vi "Initialize.vi"(8 "error in":errorcluster, 11 "cPAS Subject in":refnum<class "cPAS Subject.lvclass">) -> (0 "error out":errorcluster, 2 "DVR":refnum<data-value>, 3 "cPAS Subject out":refnum<class "cPAS Subject.lvclass">)   [LabVIEW 2015, in "cPAS Subject.lvclass"]
uses:
  cPAS Subject.lvclass
  Reusable/Data/Data.lvclass
  Data/cPAS Data.lvclass
  Reusable/Observer/Data Subject.lvclass/Data Subject.ctl
  Reusable/Observer/Data Subject.lvclass
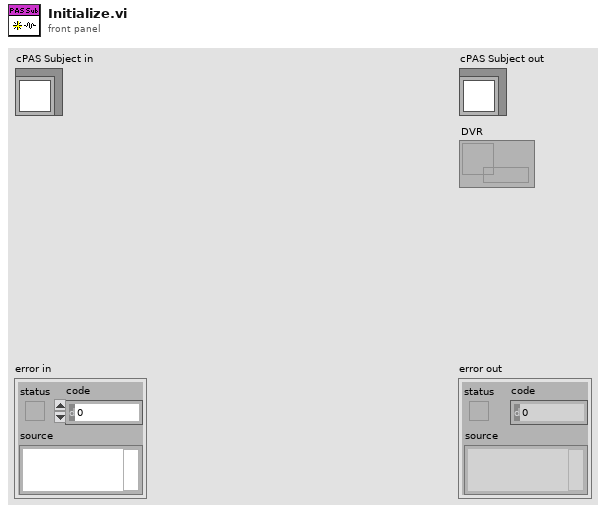
[diagram p1: front panel]
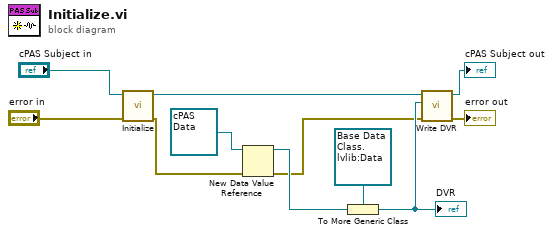
[diagram p0: block diagram]
diagram:
  n1 = call-parent "Initialize.vi"("error in"="error in", "Data Subject in"="cPAS Subject in") -> ("error out"=w8:errorcluster, "Data Subject out"=w7:refnum<class "cPAS Subject.lvclass">)  [unwired: 7 in, 1 out]
  n2 = New Data Value Reference(data value=refnum<class "cPAS Data.lvclass"> refnum ("cPAS Data"), error in=w8) -> (data value reference=w5:refnum<data-value>, error out=w1:errorcluster)
  n3 = To More Generic Class(target class=refnum<data-value> refnum ("data value reference"), reference=w5) -> (generic class reference=w3:refnum<data-value>)
  "DVR" <- w3
  n4 = call "Write DVR.vi"("error in"=w1, "DVR"=w3, "Data Subject in"=w7) -> ("error out"=→"error out":errorcluster, "Data Subject out"=→"cPAS Subject out":refnum<class "cPAS Subject.lvclass">)  [unwired: 7 in]
